vi "Disarm.vi"(8 "error in (no error)":errorcluster, 9 "Request type":T1=enum."User command", 11 "Red Pitaya Digitizer in":refnum<class "Red Pitaya Digitizer.lvclass">) -> (0 "error out":errorcluster, 2 "Armed":bool, 3 "Red Pitaya Digitizer out":refnum<class "Red Pitaya Digitizer.lvclass">)   [LabVIEW 2021, in "Red Pitaya Digitizer.lvclass"]
uses:
  LabActor/Controllers/Process Controller/Request type.ctl
  Red Pitaya Digitizer.lvclass
  Red Pitaya Digitizer.lvclass/Red Pitaya Digitizer.ctl
  Instruments/Pulse Driver/Lockin Digitizer Driver/Lockin Digitizer Driver.lvclass
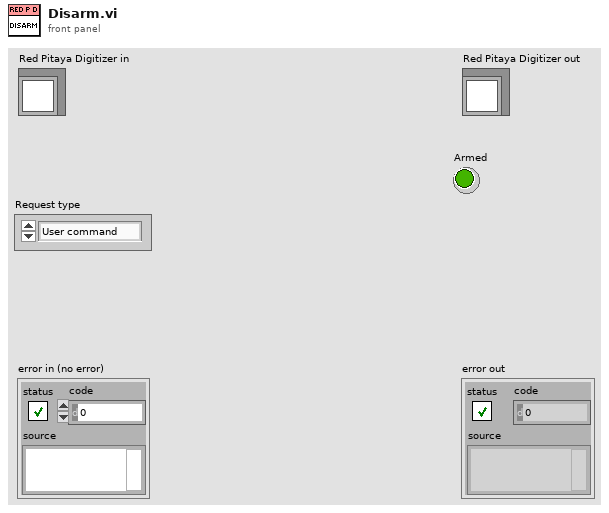
[diagram p1: front panel]
types:
  T1 = typedef "Request type.ctl" = enum16{"Process complete", "User command", "Auto-restart", "Error"}
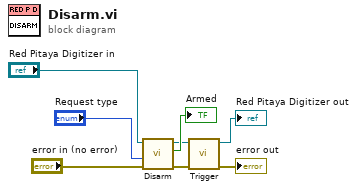
[diagram p0: block diagram]
diagram:
  n1 = call-parent "Disarm.vi"("error in (no error)"="error in (no error)", "Request type"="Request type", "Pulse Driver in"="Red Pitaya Digitizer in") -> ("error out"=w4:errorcluster, "Armed"=→"Armed":bool, "Pulse Driver out"=w3:refnum<class "Red Pitaya Digitizer.lvclass">)  [unwired: 6 in]
  n2 = call-dynamic "Trigger.vi"("error in (no error)"=w4, "Red Pitaya Digitizer in"=w3) -> ("error out"=→"error out":errorcluster, "Red Pitaya Digitizer out"=→"Red Pitaya Digitizer out":refnum<class "Red Pitaya Digitizer.lvclass">)  [unwired: 8 in]
